vi "Begin.vi"(8 "error in":errorcluster) -> (0 "error out":errorcluster)   [LabVIEW 2019]
doc: "Called before other user functions, this VI is expected to open initial I/O refnums, load in file data, and do all program initialization. Notice that the <B>error out</B> terminal is simply used for data flow. Wiring it to other structures or subVIs ensures that this VI runs first."
uses:
  <vilib>/Rock Robotics/WPI/SafetyOutput/WPI_SafetyOutputConfigMenu.ctl
  Robot Global Data.vi
  <vilib>/Rock Robotics/WPI/DriverStation/WPI_DriverStationRobotMode2.ctl
  <vilib>/Rock Robotics/WPI/Joystick/WPI_JoystickDeviceEnum.ctl
  <vilib>/Rock Robotics/WPI/MotorControl/WPI_MotorControlOpen VictorSP.vi
  <vilib>/Rock Robotics/SystemInterfaces/DIO/FPGA_DIOPWMChannel.ctl
  <vilib>/Rock Robotics/SystemInterfaces/AI/FPGA_AIChannel.ctl
  <vilib>/Rock Robotics/WPI/Switch/WPI_SwitchOpenLimit.vi
  <vilib>/Rock Robotics/SystemInterfaces/DIO/FPGA_DIOChannel.ctl
  <vilib>/Rock Robotics/WPI/Accelerometer/InternalAccelerometer/WPI_AccelerometerInternalOpen.vi
  <vilib>/Rock Robotics/WPI/Accelerometer/WPI_AccelerometerRange.ctl
  <vilib>/Rock Robotics/WPI/RobotDrive/WPI_RobotDriveOpen4MotorWithExistingMotors.vi
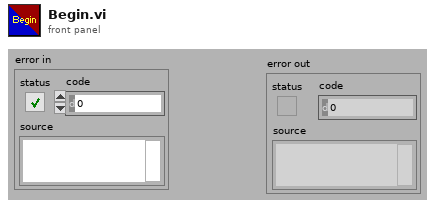
[diagram p1: front panel]
types:
  T1 = typedef "WPI_AccelerometerRange.ctl" = enum16{"+/- 2 g", "+/- 4 g", "+/- 8 g"}
  T2 = typedef "FPGA_DIOPWMChannel.ctl" = enum8{"PWM 0", "PWM 1", "PWM 2", "PWM 3", "PWM 4", "PWM 5", "PWM 6", "PWM 7", "PWM 8", "PWM 9", "PWM MXP 0", "PWM MXP 1", "PWM MXP 2", "PWM MXP 3", "PWM MXP 4", "PWM MXP 5", "PWM MXP 6", "PWM MXP 7", "PWM MXP 8", "PWM MXP 9", "Invalid"}
  T3 = typedef "FPGA_DIOChannel.ctl" = enum8{"DIO 0", "DIO 1", "DIO 2", "DIO 3", "DIO 4", "DIO 5", "DIO 6", "DIO 7", "DIO 8", "DIO 9", "DIO MXP 0", "DIO MXP 1", "DIO MXP 2", "DIO MXP 3", "DIO MXP 4", "DIO MXP 5", "DIO MXP 6", "DIO MXP 7", "DIO MXP 8", "DIO MXP 9", "DIO MXP 10", "DIO MXP 11", "DIO MXP 12", "DIO MXP 13", "DIO MXP 14", "DIO MXP 15", "SPI Port CS1", "SPI Port CS2", "SPI Port CS3", "SPI Port MISO", "SPI Port MOSI", "Invalid"}
  T4 = typedef "WPI_JoystickDeviceEnum.ctl" = enum16{"USB 0", "USB 1", "USB 2", "USB 3", "USB 4", "USB 5"}
  T5 = typedef "WPI_SafetyOutputConfigMenu.ctl" = enum16{"Enable", "Disable"}
  T6 = typedef "FPGA_AIChannel.ctl" = enum8{"AI 0", "AI 1", "AI 2", "AI 3", "AI MXP 0", "AI MXP 1", "AI MXP 2", "AI MXP 3", "Invalid"}
  T7 = typedef "WPI_DriverStationRobotMode2.ctl" = enum16{"Autonomous Disabled", "Autonomous Enabled", "Teleop Disabled", "Teleop Enabled", "Disconnected", "Finish", "Test Disabled", "Test Enabled", "Emergency Stopped"}
  T8 = typedef "WPI_MotorControlDeviceRef.ctl" = cluster{"DeviceStatus":errorcluster, "Type":T9, "PWM":cluster{"PWM Channel":T2, "DeadBand":T10}, "CAN":cluster{"Device Number":u8, "SetOutput VI Ref":variant, "GetOutput VI Ref":variant, "Enable VI Ref":variant, "Disable VI Ref":variant, "Data":variant}, "Invert":bool, "DIO PWM":cluster{"PWM \"Enable\" Channel":T2, "DIOChannel":T3, "PWM Rate":dbl}}
  T9 = typedef "WPI_MotorControlType.ctl" = enum16{"PWM", "CAN", "DIO PWM"}
  T10 = typedef "WPI_PWMDeadband.ctl" = cluster{"Name":string, "maxPositivePwm":i32, "minPositivePwm":i32, "centerPwm":i32, "maxNegativePwm":i32, "minNegativePwm":i32, "angularRange":u16}
  T11 = typedef "WPI_SwitchDevRef.ctl" = cluster{"DevStatus":errorcluster, "DIO Channel":T3, "CntIndex":T12, "Normally Closed":bool}
  T12 = typedef "FPGA_CounterCtrSystemIndex.ctl" = enum8{"Ctr 0", "Ctr 1", "Ctr 2", "Ctr 3", "Ctr 4", "Ctr 5", "Ctr 6", "Ctr 7", "Invalid"}
  T13 = typedef "WPI_ServoDeviceRef.ctl" = cluster{"DeviceStatus":errorcluster, "PWM Channel":T2, "DeadBand":T10}
  T14 = typedef "WPI_PotentiometerDevRef.ctl" = cluster{"DevStatus":errorcluster, "Analog Channel":T6, "Invert Output":bool}
  T15 = typedef "WPI_JoystickDevRef.ctl" = cluster{"Device":T4}
  T16 = typedef "WPI_RobotDriveDevRef.ctl" = cluster{"DevStatus":errorcluster, "Motors[]":T8[], "Square Inputs":bool, "Max Output":dbl}
  T17 = typedef "WPI_AccelerometerDevRef.ctl" = cluster{"DevStatus":errorcluster, "Scaling":T18, "Analog Channels":T19, "I2C Bus":T20, "SPI Bus":T21, "Accel Range":T22, "ADXL Axes":T23, "Handle":i32, "Device Address":u8, "Accel Type":enum16{"Analog", "ADXL345 I2C", "ADXL345 SPI", "Internal", "ADXL362 SPI"}}
  T18 = typedef "WPI_AccelerometerScaling.ctl" = cluster{"Gain (VoltsPerG)":dbl, "Center Voltage":dbl}
  T19 = typedef "WPI_AccelerometerAnalogChannels.ctl" = cluster{"X-Axis":T6, "Y-Axis":T6, "Z-Axis":T6}
  T20 = typedef "i2c_bus.ctl" = enum16{"I2C On-Board", "I2C MXP", "Invalid"}
  T21 = typedef "spi_bus.ctl" = enum16{"SPI On-Board, CS0", "SPI On-Board, CS1", "SPI On-Board, CS2", "SPI On-Board, CS3", "SPI MXP", "Invalid"}
  T22 = typedef "ADXL345 Range.ctl" = u8
  T23 = typedef "WPI_AccelerometerADXL345 Axes.ctl" = cluster{"X-Axis":bool, "Y-Axis":bool, "Z-Axis":bool}
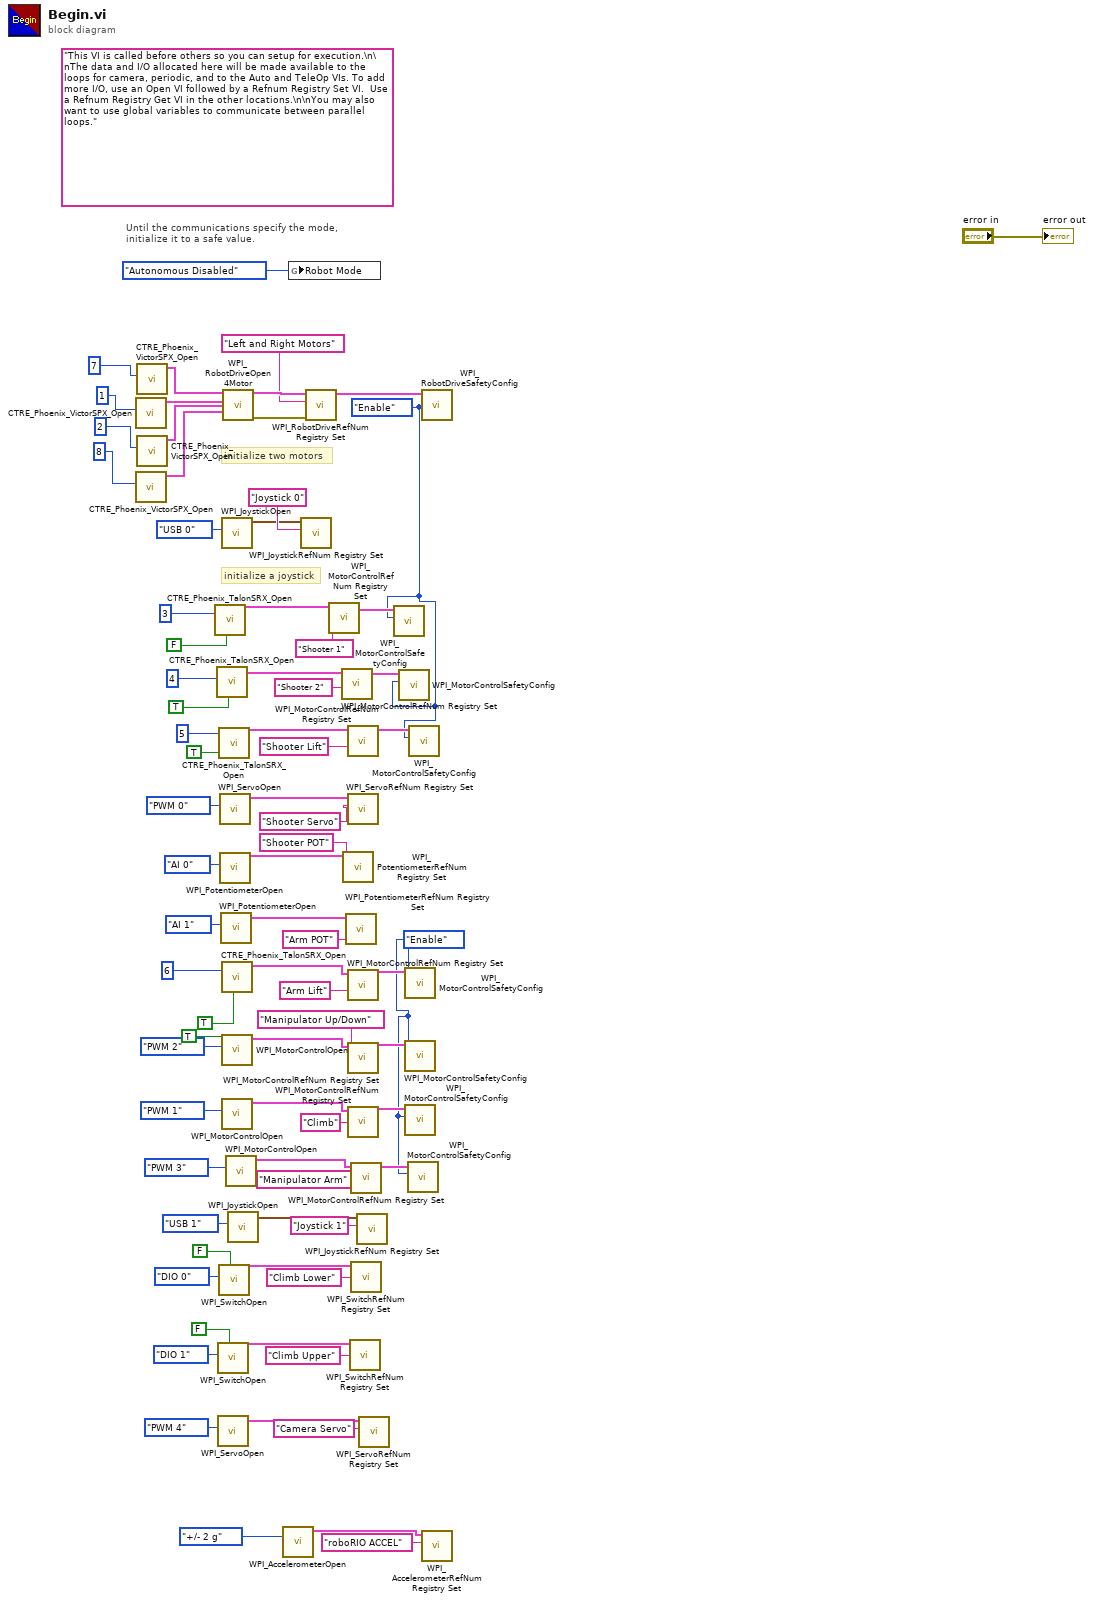
[diagram p0: block diagram]
diagram:
  w18 = WPI_SafetyOutputConfigMenu."Enable" ("mode")
  w56 = WPI_SafetyOutputConfigMenu."Enable" ("mode")
  (unwired) "This VI is called before others so you can setup for execution.\n\nThe data and I/O allocated here will be made available to the loops for camera, periodic, and to the Auto and TeleOp VIs. To add more I/O, use an Open VI followed by a Refnum Registry Set VI.  Use a Refnum Registry Get VI in the other locations.\n\nYou may also want to use global variables to communicate between parallel loops."
  # "initialize a joystick"
  # "Until the communications specify the mode,\ninitialize it to a safe value."
  # "initialize two motors"
  n1 = call <vilib>:"CTRE_Phoenix_VictorSPX_Open.vi"("Device Number"=u8 1 ("Left Motor")) -> ("CAN Talon SRX Ref"=w6:T8)  [unwired: 9 in, 1 out]
  n2 = call <vilib>:"CTRE_Phoenix_VictorSPX_Open.vi"("Device Number"=u8 8 ("Front Left Motor")) -> ("CAN Talon SRX Ref"=w4:T8)  [unwired: 9 in, 1 out]
  n3 = call <vilib>:"CTRE_Phoenix_VictorSPX_Open.vi"("Device Number"=u8 7 ("Rear Left Motor")) -> ("CAN Talon SRX Ref"=w8:T8)  [unwired: 9 in, 1 out]
  n4 = call <vilib>:"CTRE_Phoenix_VictorSPX_Open.vi"("Device Number"=u8 2 ("Right Motor")) -> ("CAN Talon SRX Ref"=w5:T8)  [unwired: 9 in, 1 out]
  n5 = call <vilib>:"CTRE_Phoenix_TalonSRX_Open.vi"("Invert"=FALSE, "Device Number"=u8 3) -> ("CAN Talon SRX Ref"=w68:T8)  [unwired: 8 in, 1 out]
  n6 = call <vilib>:"CTRE_Phoenix_TalonSRX_Open.vi"("Invert"=TRUE, "Device Number"=u8 4) -> ("CAN Talon SRX Ref"=w65:T8)  [unwired: 8 in, 1 out]
  n7 = call-poly <vilib>:"WPI_SwitchOpen.vi"("Normally Closed"=FALSE, "DIO Channel"=FPGA_DIOChannel."DIO 1") -> ("SwitchDevRef"=w20:T11)  [unwired: 8 in, 1 out]
  n8 = call <vilib>:"WPI_ServoOpen.vi"("PWM Channel"=FPGA_DIOPWMChannel."PWM 4") -> ("ServoDeviceRef"=w14:T13)  [unwired: 9 in, 1 out]
  n9 = call <vilib>:"CTRE_Phoenix_TalonSRX_Open.vi"("Invert"=TRUE, "Device Number"=u8 5) -> ("CAN Talon SRX Ref"=w63:T8)  [unwired: 8 in, 1 out]
  n10 = call-poly <vilib>:"WPI_SwitchOpen.vi"("Normally Closed"=FALSE, "DIO Channel"=FPGA_DIOChannel."DIO 0") -> ("SwitchDevRef"=w27:T11)  [unwired: 8 in, 1 out]
  n11 = call <vilib>:"WPI_ServoOpen.vi"("PWM Channel"=FPGA_DIOPWMChannel."PWM 0") -> ("ServoDeviceRef"=w60:T13)  [unwired: 9 in, 1 out]
  n12 = call <vilib>:"WPI_PotentiometerOpen.vi"("Analog Channel"=FPGA_AIChannel."AI 0") -> ("PotDevRef"=w53:T14)  [unwired: 9 in, 1 out]
  n13 = call <vilib>:"WPI_PotentiometerOpen.vi"("Analog Channel"=FPGA_AIChannel."AI 1") -> ("PotDevRef"=w48:T14)  [unwired: 9 in, 1 out]
  n14 = call <vilib>:"WPI_JoystickOpen.vi"("JoystickDevice"=WPI_JoystickDeviceEnum."USB 0") -> ("JoystickDevRef"=w72:T15)  [unwired: 10 in]
  n15 = call <vilib>:"CTRE_Phoenix_TalonSRX_Open.vi"("Invert"=TRUE, "Device Number"=u8 6) -> ("CAN Talon SRX Ref"=w45:T8)  [unwired: 8 in, 1 out]
  n16 = call-poly <vilib>:"WPI_MotorControlOpen.vi"("Eliminate Deadband"=TRUE, "PWM Channel"=FPGA_DIOPWMChannel."PWM 2") -> ("MotorControlDeviceRef"=w38:T8)  [unwired: 8 in, 1 out]
  n17 = call-poly <vilib>:"WPI_MotorControlOpen.vi"("PWM Channel"=FPGA_DIOPWMChannel."PWM 1") -> ("MotorControlDeviceRef"=w37:T8)  [unwired: 9 in, 1 out]
  n18 = call-poly <vilib>:"WPI_RobotDriveOpen4Motor.vi"("Rear Left Motor Dev Ref"=w8, "Rear Right Motor Dev Ref"=w6, "Front Left Motor Dev Ref"=w5, "Front Right Motor Dev Ref"=w4) -> ("RobotDriveDevRef"=w78:T16, "error out"=w76:errorcluster)  [unwired: 10 in]
  n19 = call-poly <vilib>:"WPI_MotorControlOpen.vi"("PWM Channel"=FPGA_DIOPWMChannel."PWM 3") -> ("MotorControlDeviceRef"=w17:T8)  [unwired: 9 in, 1 out]
  n20 = call <vilib>:"WPI_JoystickOpen.vi"("JoystickDevice"=WPI_JoystickDeviceEnum."USB 1") -> ("JoystickDevRef"=w33:T15)  [unwired: 10 in]
  n21 = call-poly <vilib>:"WPI_AccelerometerOpen.vi"("Accel Range"=WPI_AccelerometerRange."+/- 2 g") -> ("AccelerometerDevRef"=w11:T17)  [unwired: 9 in, 1 out]
  n22 = global write "Robot Global Data.vi" "Robot Mode"(WPI_DriverStationRobotMode2."Autonomous Disabled" ("Robot Mode")) -> ()
  n23 = call <vilib>:"WPI_JoystickRefNum Registry Set.vi"("refnum name"="Joystick 0", "JoystickDevRef"=w72) -> ()  [unwired: 8 in, 2 out]
  n24 = call <vilib>:"WPI_RobotDriveRefNum Registry Set.vi"("error in (no error)"=w76, "refnum name"="Left and Right Motors", "RobotDriveDevRef"=w78) -> ("RobotDriveDevRef"=w75:T16)  [unwired: 1 in, 7 out]
  n25 = call <vilib>:"WPI_MotorControlRefNum Registry Set.vi"("refnum name"="Shooter 1", "MotorControlDevRef"=w68) -> ("MotorControlDevRef"=w59:T8)  [unwired: 8 in, 1 out]
  n26 = call <vilib>:"WPI_MotorControlRefNum Registry Set.vi"("refnum name"="Shooter 2", "MotorControlDevRef"=w65) -> ("MotorControlDevRef"=w58:T8)  [unwired: 8 in, 1 out]
  n27 = call <vilib>:"WPI_PotentiometerRefNum Registry Set.vi"("refnum name"="Shooter POT", "PotDevRef"=w53) -> ()  [unwired: 8 in, 2 out]
  n28 = call <vilib>:"WPI_PotentiometerRefNum Registry Set.vi"("refnum name"="Arm POT", "PotDevRef"=w48) -> ()  [unwired: 8 in, 2 out]
  n29 = call <vilib>:"WPI_MotorControlRefNum Registry Set.vi"("refnum name"="Shooter Lift", "MotorControlDevRef"=w63) -> ("MotorControlDevRef"=w57:T8)  [unwired: 8 in, 1 out]
  n30 = call <vilib>:"WPI_ServoRefNum Registry Set.vi"("refnum name"="Shooter Servo", "ServoDeviceRef"=w60) -> ()  [unwired: 8 in, 2 out]
  n31 = call <vilib>:"WPI_MotorControlRefNum Registry Set.vi"("refnum name"="Arm Lift", "MotorControlDevRef"=w45) -> ("MotorControlDevRef"=w42:T8)  [unwired: 8 in, 1 out]
  n32 = call <vilib>:"WPI_MotorControlRefNum Registry Set.vi"("refnum name"="Manipulator Up/Down", "MotorControlDevRef"=w38) -> ("MotorControlDevRef"=w41:T8)  [unwired: 8 in, 1 out]
  n33 = call <vilib>:"WPI_MotorControlRefNum Registry Set.vi"("refnum name"="Climb", "MotorControlDevRef"=w37) -> ("MotorControlDevRef"=w34:T8)  [unwired: 8 in, 1 out]
  n34 = call <vilib>:"WPI_SwitchRefNum Registry Set.vi"("refnum name"="Climb Upper", "SwitchDevRef"=w20) -> ()  [unwired: 8 in, 2 out]
  n35 = call <vilib>:"WPI_MotorControlRefNum Registry Set.vi"("refnum name"="Manipulator Arm", "MotorControlDevRef"=w17) -> ("MotorControlDevRef"=w19:T8)  [unwired: 8 in, 1 out]
  n36 = call <vilib>:"WPI_SwitchRefNum Registry Set.vi"("refnum name"="Climb Lower", "SwitchDevRef"=w27) -> ()  [unwired: 8 in, 2 out]
  n37 = call <vilib>:"WPI_JoystickRefNum Registry Set.vi"("refnum name"="Joystick 1", "JoystickDevRef"=w33) -> ()  [unwired: 8 in, 2 out]
  n38 = call <vilib>:"WPI_ServoRefNum Registry Set.vi"("refnum name"="Camera Servo", "ServoDeviceRef"=w14) -> ()  [unwired: 8 in, 2 out]
  n39 = call <vilib>:"WPI_MotorControlSafetyConfig.vi"("mode"=w56, "MotorControlDevRef"=w59) -> ()  [unwired: 8 in, 2 out]
  n40 = call <vilib>:"WPI_MotorControlSafetyConfig.vi"("mode"=w56, "MotorControlDevRef"=w58) -> ()  [unwired: 8 in, 2 out]
  n41 = call <vilib>:"WPI_MotorControlSafetyConfig.vi"("mode"=w18, "MotorControlDevRef"=w42) -> ()  [unwired: 8 in, 2 out]
  n42 = call <vilib>:"WPI_MotorControlSafetyConfig.vi"("mode"=w18, "MotorControlDevRef"=w41) -> ()  [unwired: 8 in, 2 out]
  n43 = call <vilib>:"WPI_MotorControlSafetyConfig.vi"("mode"=w18, "MotorControlDevRef"=w34) -> ()  [unwired: 8 in, 2 out]
  n44 = call <vilib>:"WPI_MotorControlSafetyConfig.vi"("mode"=w18, "MotorControlDevRef"=w19) -> ()  [unwired: 8 in, 2 out]
  n45 = call <vilib>:"WPI_MotorControlSafetyConfig.vi"("mode"=w56, "MotorControlDevRef"=w57) -> ()  [unwired: 8 in, 2 out]
  n46 = call <vilib>:"WPI_RobotDriveSafetyConfig.vi"("mode"=w56, "RobotDriveDevRef"=w75) -> ()  [unwired: 8 in, 2 out]
  n47 = call <vilib>:"WPI_AccelerometerRefNum Registry Set.vi"("refnum name"="roboRIO ACCEL", "AccelerometerDevRef"=w11) -> ()  [unwired: 8 in, 2 out]
  "error out" <- "error in"
